vi "AuMT8852B Tester Rear Panel Output.vi"(5 "Rear Panel Settings":T2, 7 "Set/Get (Set)":enum16{"Set", "Get"}(ring), 8 "error in (no error)":errorcluster, 11 "VISA session":refnum<visa-resource-name>) -> (0 "error out":errorcluster, 2 "error code":i32, 3 "VISA session out":refnum<visa-resource-name>, 4 "Rear Panel Settings out":T1)   [LabVIEW 2017]
doc: "Anritsu MT8852B Bluetooth Tester\n\nDefines the output directed to the rear panel BNC outputs.\n\nThe allowable selections are restricted as follows:\n- Output 1 cannot be RXON and Output 2 cannot be TXON.\n- If Output 1 is TXON, Output 2 can be any value.\n- If Output 2 is RXON, Output 1 can be any value.\n- Otherwise Output 1 and Output 2 must be set to the same value.\n\nINPUTS\nSet/Get - whether the value is being sent to or retrieved from the instrument.\nRear Panel Settings - the output settings according to the allowed combinations.\n\nOUTPUTS\nRear Panel Settings out - the BNC output settings currently in use."
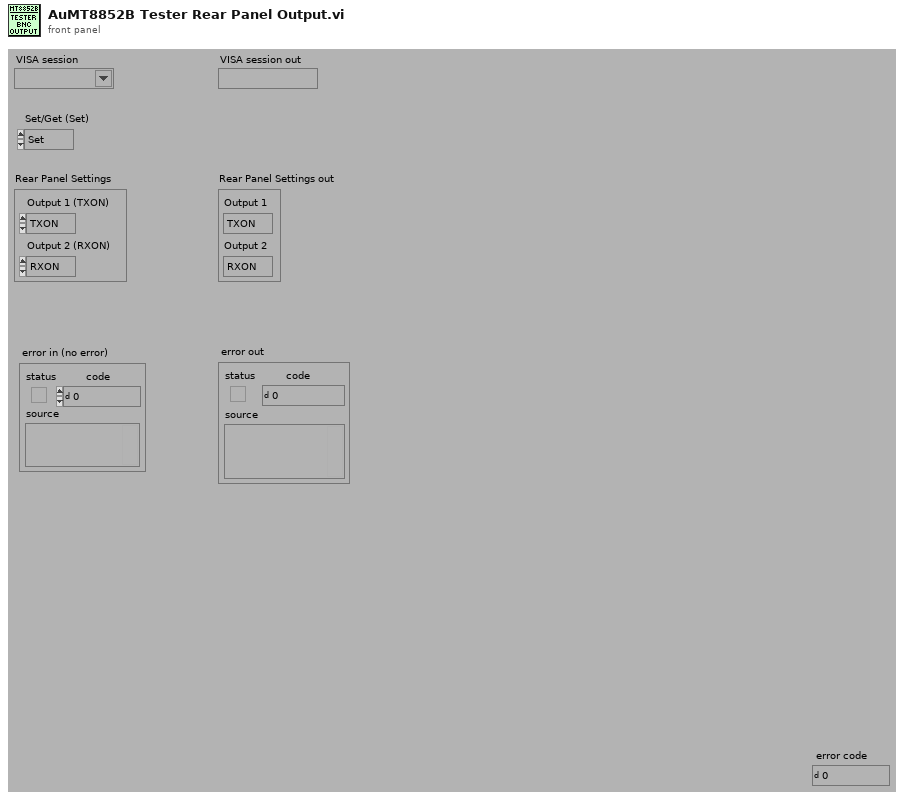
[diagram p1: front panel]
types:
  T1 = cluster{"Output 2":enum16{"RXON", "RXDATA", "CORRFIRED"}, "Output 1":enum16{"TXON", "RXDATA", "CORRFIRED"}}
  T2 = cluster{"Output 2 (RXON)":enum16{"RXON", "RXDATA", "CORRFIRED"}, "Output 1 (TXON)":enum16{"TXON", "RXDATA", "CORRFIRED"}}
  T3 = enum16{"Simulate", "Range check", "Cache", "Query instrument status"}
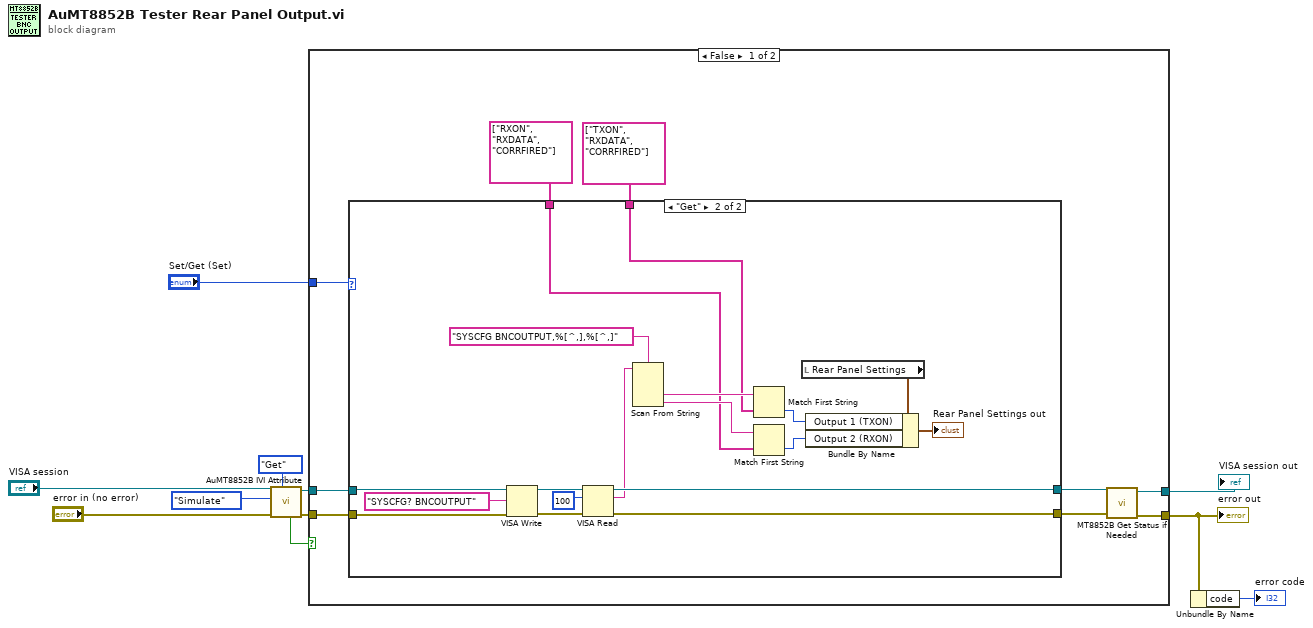
[diagram p0: block diagram]
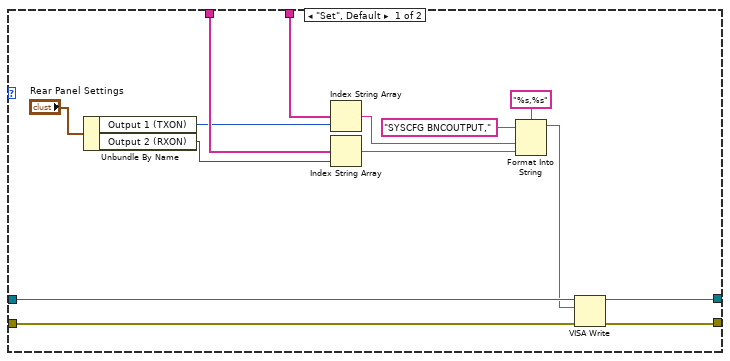
[diagram p2: hidden frame]
diagram:
  n1 = call <instrlib>:"AuMT8852B IVI Attribute.vi"("Set/Get (Set)"=enum16{"Set", "Get"}."Get", "error in (no error)"="error in (no error)", "Flag (Simulate)"=T3."Simulate", "VISA session"="VISA session") -> ("error out"=w9:errorcluster, "VISA session out"=w8:refnum<visa-resource-name>, "Value out"=w10:bool)  [unwired: 5 in]
  n2 = case shown="False" w10 {
    tunnel: [w19 w53] -> w6
    tunnel: [w20 w54] -> w1
    tunnel: "Set/Get (Set)" -> [w16 _]
    tunnel: w9 -> [w15 w54]
    tunnel: w8 -> [w14 w53]
    frame False {
      n3 = case shown="\"Get\"" w16 {
        tunnel: [w32 w45] -> w17
        tunnel: [w31 w44] -> w18
        tunnel: w15 -> [w34 w49]
        tunnel: w14 -> [w33 w48]
        tunnel: string[] ["RXON", "RXDATA", "CORRFIRED"] -> [w26 w39]
        tunnel: string[] ["TXON", "RXDATA", "CORRFIRED"] -> [w24 w40]
        frame "Set", Default {
          n4 = Unbundle By Name("Rear Panel Settings") -> ("Output 1 (TXON)"=w22:enum16{"TXON", "RXDATA", "CORRFIRED"}, "Output 2 (RXON)"=w21:enum16{"RXON", "RXDATA", "CORRFIRED"})
          n5 = Index String Array(1:w22, 2:w24) -> (0:w25:string)  [unwired: 1 in]
          n6 = Index String Array(1:w21, 2:w26) -> (0:w27:string)  [unwired: 1 in]
          n7 = Format Into String(format string="%s,%s", initial string="SYSCFG BNCOUTPUT,", w25, w27) -> (resulting string=w28:string)  [unwired: 1 in, 1 out]
          n8 = VISA Write(VISA resource name=w33, write buffer=w28, error in (no error)=w34) -> (VISA resource name out=w32:refnum<visa-resource-name>, error out=w31:errorcluster)  [unwired: 1 out]
        }
        frame "Get" {
          n9 = VISA Write(VISA resource name=w48, write buffer="SYSCFG? BNCOUTPUT", error in (no error)=w49) -> (VISA resource name out=w51:refnum<visa-resource-name>, error out=w52:errorcluster)  [unwired: 1 out]
          n10 = VISA Read(VISA resource name=w51, byte count=u32 100 ("byte count (0)"), error in (no error)=w52) -> (VISA resource name out=w45:refnum<visa-resource-name>, read buffer=w43:string, error out=w44:errorcluster)  [unwired: 1 out]
          n11 = Scan From String(format string="SYSCFG BNCOUTPUT,%[^,],%[^,]", input string=w43) -> (output 1=w42:string, output 2=w41:string)  [unwired: 4 in, 3 out]
          n12 = Match First String(2:w40, 3:w42) -> (0:w37:i32)  [unwired: 1 out]
          n13 = Match First String(2:w39, 3:w41) -> (0:w38:i32)  [unwired: 1 out]
          n14 = local read "Rear Panel Settings"() -> (w36:T2)
          n15 = Bundle By Name(cluster=w36, "Output 1 (TXON)"=w37, "Output 2 (RXON)"=w38) -> (→"Rear Panel Settings out":T2)
        }
      }
      n16 = call <instrlib>:"MT8852B Get Status if Needed.vi"("error in (no error)"=w18, "VISA session"=w17) -> ("error out"=w20:errorcluster, "VISA session out"=w19:refnum<visa-resource-name>)  [unwired: 8 in]
    }
    frame True {
    }
  }
  "VISA session out" <- w6
  "error out" <- w1
  n17 = Unbundle By Name(w1) -> ("code"=→"error code":i32)
